vi "p4_banda.vi"() -> ()   [LabVIEW 2019]
panel:
  in  "stop":bool
  in  "Direccion":bool
  in  "Velocidad(1m/300ms)":sgl(knob) scale=0.0..10.0
  out "Slide":sgl(slide) scale=0.0..1200.0
  # "Derecha"
  # "Izquierda"
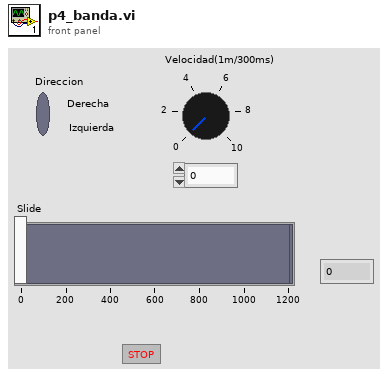
[diagram p1: front panel]
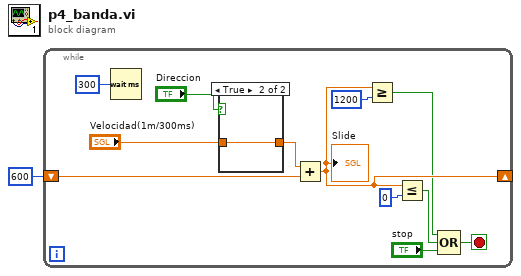
[diagram p0: block diagram]
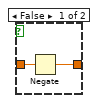
[diagram p2: hidden frame]
diagram:
  n1 = while {
    shift-right: [w6] -> _
    shift-left: i16 600 -> [w10]
    stop <- w2 stop-if-true
    n2 = Wait (ms)(milliseconds to wait=i16 300) -> ()  [unwired: 1 out]
    n3 = case shown="True" "Direccion" {
      tunnel: "Velocidad(1m/300ms)" -> [w15 w16]
      tunnel: [w14 w16] -> w11
      frame False {
        n4 = Negate(x=w15) -> (-x=w14:sgl)
      }
      frame True {
      }
    }
    n5 = Add(x=w11, y=w10) -> (x+y=w6:sgl)
    "Slide" <- w6
    n6 = Greater Or Equal?(x=w6, y=u16 1200) -> (x >= y?=w5:bool)
    n7 = Less Or Equal?(x=w6, y=u8 0) -> (x <= y?=w4:bool)
    n8 = Compound Arithmetic op=OR(w5, w4, "stop") -> (w2:bool)
  }
